vi "Init.vi"(8 "error in (no error)":errorcluster, 10 "Node Reg":refnum<k20>, 11 "MultiDiagramStructure in":refnum<class "MultiDiagramStructure.lvclass">) -> (0 "error out":errorcluster, 3 "MultiDiagramStructure out":refnum<class "MultiDiagramStructure.lvclass">)   [LabVIEW 2021, in "MultiDiagramStructure.lvclass"]
uses:
  MultiDiagramStructure.lvclass
  Subdiagram.ctl
  Node/Node.lvclass
  <vilib>/xml/NI_XML.lvlib
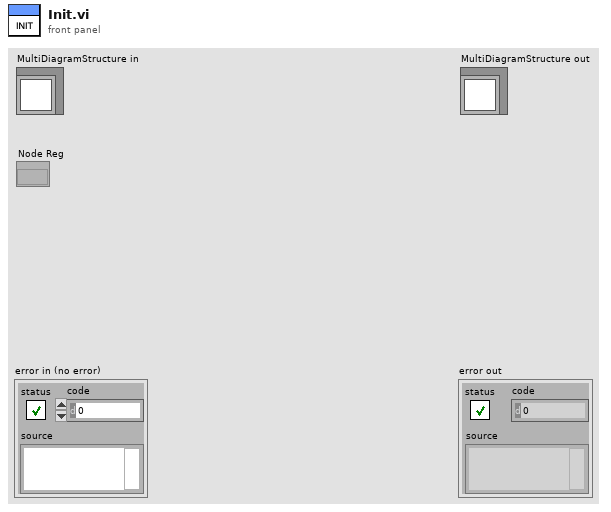
[diagram p1: front panel]
types:
  T1 = typedef "Subdiagram.ctl" = cluster{"diagram":refnum<vi>, "selector":string, "uuid":string}
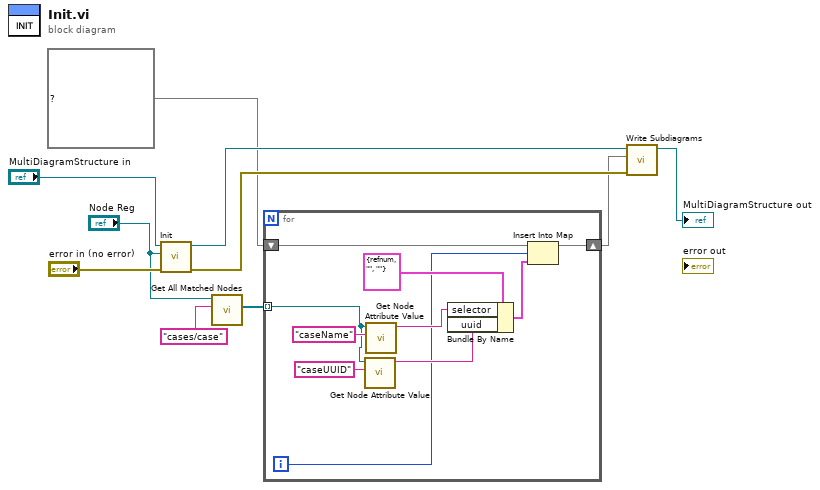
[diagram p0: block diagram]
diagram:
  n1 = call-parent "Init.vi"("error in (no error)"="error in (no error)", "Node Reg"="Node Reg", "Node in"="MultiDiagramStructure in") -> ("error out"=w3:errorcluster, "Node out"=w5:refnum<class "MultiDiagramStructure.lvclass">)  [unwired: 7 in]
  n2 = call <vilib>:"Get All Matched Nodes.vi"("XPath expression"="cases/case", "node in"="Node Reg") -> ("node result array"=w6:refnum<k20>[])  [unwired: 7 in, 2 out]
  n3 = for {
    tunnel: w6 -> [w18] mode=indexing
    shift-right: [w16] -> w1
    shift-left: map{u64, T1} {} ("Subdiagrams") -> [w17]
    i -> [w11]
    n4 = call "Get Node Attribute Value.vi"("Attribute Name"="caseUUID", "Refnum in"=w18) -> ("Value"=w12:string)  [unwired: 9 in]
    n5 = call "Get Node Attribute Value.vi"("Attribute Name"="caseName", "Refnum in"=w18) -> ("Value"=w13:string)  [unwired: 9 in]
    n6 = Bundle By Name(cluster=T1 {"diagram"=refnum, "selector"="", "uuid"=""} ("value"), "selector"=w13, "uuid"=w12) -> (w14:T1)
    n7 = Insert Into Map(map in=w17, key=w11, value=w14) -> (map out=w16:map{u64, T1})  [unwired: 2 out]
  }
  n8 = call-dynamic "Write Subdiagrams.vi"("error in (no error)"=w3, "Subdiagrams"=w1, "MultiDiagramStructure in"=w5) -> ("MultiDiagramStructure out"=→"MultiDiagramStructure out":refnum<class "MultiDiagramStructure.lvclass">)  [unwired: 7 in, 1 out]
